vi "Read (Digitize).vi"(0 "VISA resource name":refnum<visa-resource-name>="USB0::0x05E6::0x2461::04090176::INSTR", 5 "Timeout (10000 ms)":i32=10000 format="%#.6g", 7 "Buffer Name (defbuffer1)":string="defbuffer1", 9 "Buffer Elements":string="READ", 11 "error in (no error)":errorcluster) -> (4 "VISA resource name out":refnum<visa-resource-name>="USB0::0x05E6::0x2461::04090176::INSTR", 6 "Data out":string="-7.913777E+01\n", 15 "error out":errorcluster)   [LabVIEW 2018, in "Keithley 2450.lvlib"]
doc: "This query makes a digitize measurement, places it in a reading buffer, and returns the latest reading.\n\nYou must set the instrument to a digitize function before sending this command.\nThis query makes the number of readings specified by [:SENSe[1]]:DIGitize:COUNt. If multiple\nreadings are made, all readings are available in the reading buffer. However, only the last reading is\nreturned as a reading with the command. To get multiple readings, use the :TRACe:DATA?\ncommand.\nWhen specifying buffer elements, you can:\n• Specify buffer elements in any order.\n• Include any or all of the buffer elements listed below in a single list. You can repeat elements as\nlong as the number of elements in the list is less than 14.\n• Use a comma to delineate multiple elements for a data point.\n\n<B>This function is only compatible with the 2461.</B>"
uses:
  <instrlib>/Keithley 2450/Keithley 2450.lvlib
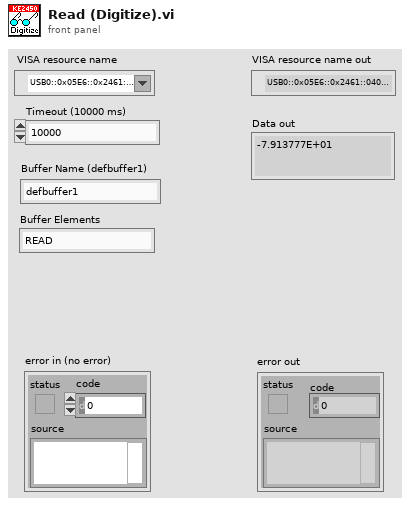
[diagram p1: front panel]
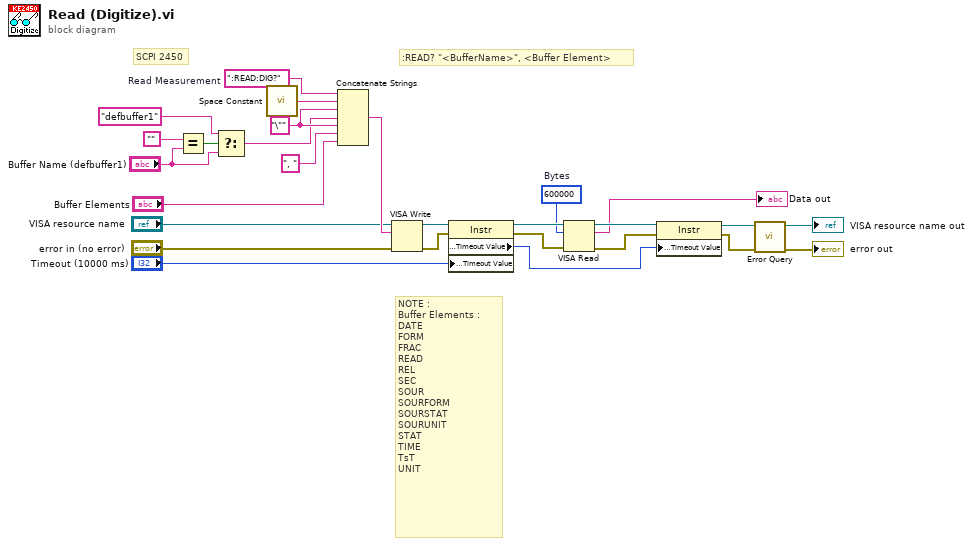
[diagram p0: block diagram]
diagram:
  w12 = "\""
  w9 = ":READ:DIG?"  # Read Measurement
  w19 = u32 600000  # Bytes
  # "NOTE :\nBuffer Elements :\nDATE\nFORM\nFRAC\nREAD\nREL\nSEC\nSOUR\nSOURFORM\nSOURSTAT\nSOURUNIT\nSTAT\nTIME\nTsT\nUNIT"
  # ":READ? \"<BufferName>\", <Buffer Element>"
  # "SCPI 2450"
  n1 = Equal?(x="", y="Buffer Name (defbuffer1)") -> (x = y?=w15:bool)
  n2 = Select(t="defbuffer1", s=w15, f="Buffer Name (defbuffer1)") -> (s? t:f=w11:string)
  n3 = call <vilib>:"Space Constant.vi"() -> ("String"=w10:string)
  n4 = Concatenate Strings(w9, w10, w12, w11, w12, ", " ("string"), "Buffer Elements") -> (w26:string)
  n5 = VISA Write(VISA resource name="VISA resource name", write buffer=w26, error in (no error)="error in (no error)") -> (VISA resource name out=w17:refnum<visa-resource-name>, error out=w25:errorcluster)  [unwired: 1 out]
  n6 = property class="Instr"(reference=w17, error in=w25, "General Settings:Timeout Value"="Timeout (10000 ms)") -> (reference out=w24:refnum<visa-resource-name>, error out=w23:errorcluster, "General Settings:Timeout Value"=w20:u32)
  n7 = VISA Read(VISA resource name=w24, byte count=w19, error in (no error)=w23) -> (VISA resource name out=w22:refnum<visa-resource-name>, read buffer=→"Data out":string, error out=w21:errorcluster)  [unwired: 1 out]
  n8 = property class="Instr"(reference=w22, error in=w21, "General Settings:Timeout Value"=w20) -> (reference out=w5:refnum<visa-resource-name>, error out=w4:errorcluster)
  n9 = call <instrlib>:"Error Query.vi"("error in (no error)"=w4, "VISA resource name"=w5) -> ("error out"=→"error out":errorcluster, "VISA resource name out"=→"VISA resource name out":refnum<visa-resource-name>)  [unwired: 8 out]
